vi "Get Mode Status.vi"(0 "VISA resource name":refnum<visa-resource-name>, 11 "error in (no error)":errorcluster) -> (2 "Single Step Mode Status":bool, 3 "Step Connect Mode Status":bool, 4 "VISA resource name out":refnum<visa-resource-name>, 6 "Voltage Range Mode":u16(ring) items=["High", "Auto"], 8 "Over Current Fold Back Mode Status":bool, 10 "Surge Drop Mode Status":bool caption="SD Mode Status", 14 "SD Continuous Mode Status":bool, 15 "error out":errorcluster)   [LabVIEW 2016, in "APT 300XAC Series.lvlib"]
doc: "Gets the Status of the various modes available in the instrument.\nReturns the status of the following modes\n\nNote : Can be used in <B>Program Mode</B> only.\n\n1. Single Step Mode\n2. Step Connect Mode\n3. Voltage Range Mode\n4. Over Current Fold Back Mode\n5. Surge Drop Mode\n6. Surge Drop Continuous Mode"
uses:
  APT 300XAC Series.lvlib
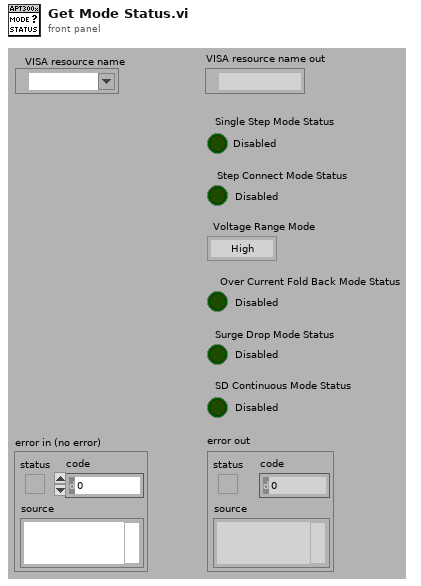
[diagram p1: front panel]
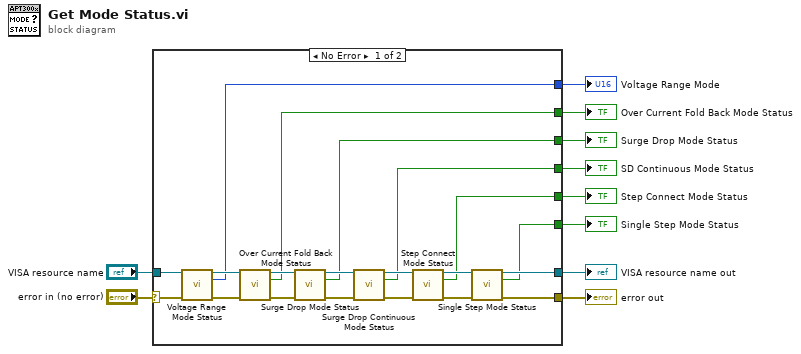
[diagram p0: block diagram]
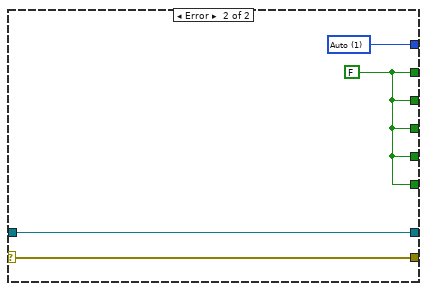
[diagram p2: hidden frame]
diagram:
  n1 = case shown="No Error" "error in (no error)" {
    selector: "error in (no error)" -> [w11 w34]
    tunnel: "VISA resource name" -> [w30 w33]
    tunnel: [w24 w33] -> w9
    tunnel: [w23 w34] -> w8
    tunnel: [w17 w31] -> w7
    tunnel: [w16 w31] -> w6
    tunnel: [w15 w31] -> w5
    tunnel: [w14 w31] -> w4
    tunnel: [w13 w31] -> w3
    tunnel: [w12 w32] -> w2
    frame No Error {
      n2 = call "Voltage Range Mode Status.vi"("VISA resource name"=w30, "error in (no error)"=w11) -> ("VISA resource name out"=w29:refnum<visa-resource-name>, "Voltage Range Mode"=w12:u16, "error out"=w18:errorcluster)  [unwired: 11 in]
      n3 = call "Over Current Fold Back Mode Status.vi"("VISA resource name"=w29, "error in (no error)"=w18) -> ("VISA resource name out"=w28:refnum<visa-resource-name>, "Over Current Fold Back Mode Status"=w13:bool, "error out"=w19:errorcluster)  [unwired: 11 in]
      n4 = call "Surge Drop Mode Status.vi"("VISA resource name"=w28, "error in (no error)"=w19) -> ("VISA resource name out"=w27:refnum<visa-resource-name>, "Surge Drop Mode Status"=w14:bool, "error out"=w20:errorcluster)  [unwired: 11 in]
      n5 = call "Surge Drop Continuous Mode Status.vi"("VISA resource name"=w27, "error in (no error)"=w20) -> ("VISA resource name out"=w26:refnum<visa-resource-name>, "SD Continuous Mode Status"=w15:bool, "error out"=w21:errorcluster)  [unwired: 11 in]
      n6 = call "Step Connect Mode Status.vi"("VISA resource name"=w26, "error in (no error)"=w21) -> ("VISA resource name out"=w25:refnum<visa-resource-name>, "Step Connect Mode Status"=w16:bool, "error out"=w22:errorcluster)  [unwired: 11 in]
      n7 = call "Single Step Mode Status.vi"("VISA resource name"=w25, "error in (no error)"=w22) -> ("VISA resource name out"=w24:refnum<visa-resource-name>, "Single Step Mode Status"=w17:bool, "error out"=w23:errorcluster)  [unwired: 11 in]
    }
    frame Error {
      w32 = u16 1 items=["High", "Auto"] ("Voltage Range Mode")
      w31 = FALSE ("Over Current Fold Back Mode Status")
    }
  }
  "VISA resource name out" <- w9
  "error out" <- w8
  "Single Step Mode Status" <- w7
  "Step Connect Mode Status" <- w6
  "SD Continuous Mode Status" <- w5
  "Surge Drop Mode Status" <- w4
  "Over Current Fold Back Mode Status" <- w3
  "Voltage Range Mode" <- w2
